vi "LoadItemValuesFromFile.vi"(0 "Array in":string[][](array[string]), 11 "error in (no error)":errorcluster) -> (3 "Values":dbl[](array[numeric]), 4 "Item":string, 6 "ZoomAlarmArray":dbl[][](array[numeric]), 8 "TimeString":string[](array[string]), 10 "TimeStamp":dbl[](array[numeric]), 13 "AlarmChannelNames":string[](array[string]), 14 "AlarmWaveforms":waveform(dbl)[](array[waveform]), 15 "error out":errorcluster)   [LabVIEW 2018]
doc: "Each row of the input string array specifies the Item, Dataset, Group, and Filepath of the data to be queried.\nUse these strings to look up the relevant data within the HDF5 records. The output values and corresponding TimeString or Timestamp arrays are suitable for plotting.\n\nItem (MaxValue, PeakLoc, etc.)\nDataset (Beac, Cal, etc.)\nGroup (84GHz_Cross, 72GHz_Cross, etc.)\nFile (filename of the HDF5 file)"
uses:
  HDF5/AI_alarm_data_cluster.ctl
  HDF5/HDF5_TC_Errors.ctl
  HDF5/TC_Data_Structure.ctl
  HDF5/HDF5_ToneInfoClust.ctl
  <vilib>/addons/h5labview2/file/H5Fmode.ctl
  HDF5/lib_path_mod_20200519.vi
  <vilib>/addons/h5labview2/base/H5Equery.vi
  <vilib>/addons/h5labview2/dataset/H5Dread.llb/H5Dread.xnode
  <vilib>/addons/h5labview2/file/H5F.lvlib
  <vilib>/addons/h5labview2/group/H5G.lvlib
  <vilib>/addons/h5labview2/dataset/H5D.lvlib
panel:
  in  "HDF5_TCInfo":T1
  in  "TC_alarm":T2
  in  "AI_alarm_Clust":T3
  # "Item"
  # "Dataset"
  # "Group"
  # "Filepath"
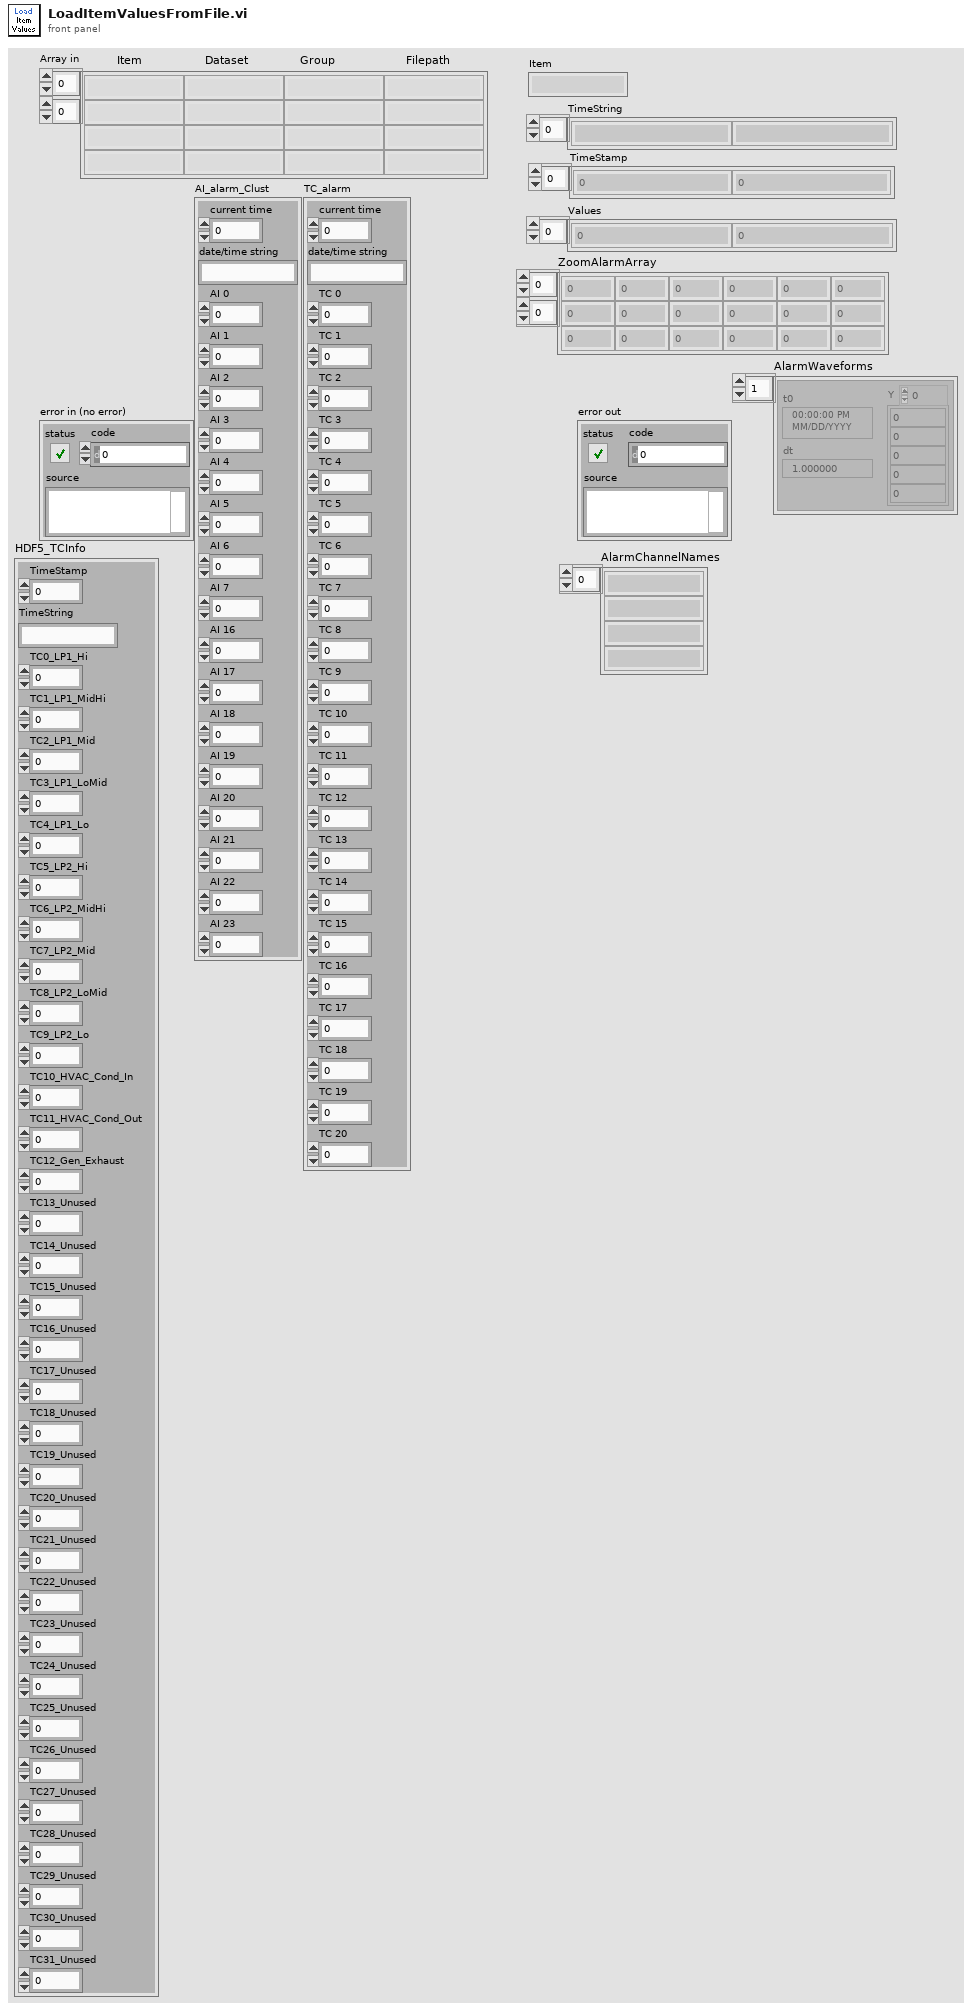
[diagram p1: front panel]
types:
  T1 = typedef "TC_Data_Structure.ctl" = cluster{"TimeStamp":dbl, "TimeString":string, "TC0_LP1_Hi":dbl, "TC1_LP1_MidHi":dbl, "TC2_LP1_Mid":dbl, "TC3_LP1_LoMid":dbl, "TC4_LP1_Lo":dbl, "TC5_LP2_Hi":dbl, "TC6_LP2_MidHi":dbl, "TC7_LP2_Mid":dbl, "TC8_LP2_LoMid":dbl, "TC9_LP2_Lo":dbl, "TC10_HVAC_Cond_In":dbl, "TC11_HVAC_Cond_Out":dbl, "TC12_Gen_Exhaust":dbl, "TC13_Unused":dbl, "TC14_Unused":dbl, "TC15_Unused":dbl, "TC16_Unused":dbl, "TC17_Unused":dbl, "TC18_Unused":dbl, "TC19_Unused":dbl, "TC20_Unused":dbl, "TC21_Unused":dbl, "TC22_Unused":dbl, "TC23_Unused":dbl, "TC24_Unused":dbl, "TC25_Unused":dbl, "TC26_Unused":dbl, "TC27_Unused":dbl, "TC28_Unused":dbl, "TC29_Unused":dbl, "TC30_Unused":dbl, "TC31_Unused":dbl}
  T2 = typedef "HDF5_TC_Errors.ctl" = cluster{"current time":dbl, "date/time string":string, "TC 0":dbl, "TC 1":dbl, "TC 2":dbl, "TC 3":dbl, "TC 4":dbl, "TC 5":dbl, "TC 6":dbl, "TC 7":dbl, "TC 8":dbl, "TC 9":dbl, "TC 10":dbl, "TC 11":dbl, "TC 12":dbl, "TC 13":dbl, "TC 14":dbl, "TC 15":dbl, "TC 16":dbl, "TC 17":dbl, "TC 18":dbl, "TC 19":dbl, "TC 20":dbl}
  T3 = typedef "AI_alarm_data_cluster.ctl" = cluster{"current time":dbl, "date/time string":string, "AI 0":dbl, "AI 1":dbl, "AI 2":dbl, "AI 3":dbl, "AI 4":dbl, "AI 5":dbl, "AI 6":dbl, "AI 7":dbl, "AI 16":dbl, "AI 17":dbl, "AI 18":dbl, "AI 19":dbl, "AI 20":dbl, "AI 21":dbl, "AI 22":dbl, "AI 23":dbl}
  T4 = typedef "H5F.lvlib/H5Fmode.ctl" = enum16{"read-only", "read-write", "overwrite", "create new", "open or create"}
  T5 = typedef "HDF5_ToneInfoClust.ctl" = cluster{"Timestring":string, "Timestamp":dbl, "MaxValue":dbl, "PeakLoc":dbl, "df":dbl}
  T6 = typedef "hid_t.ctl" = i32
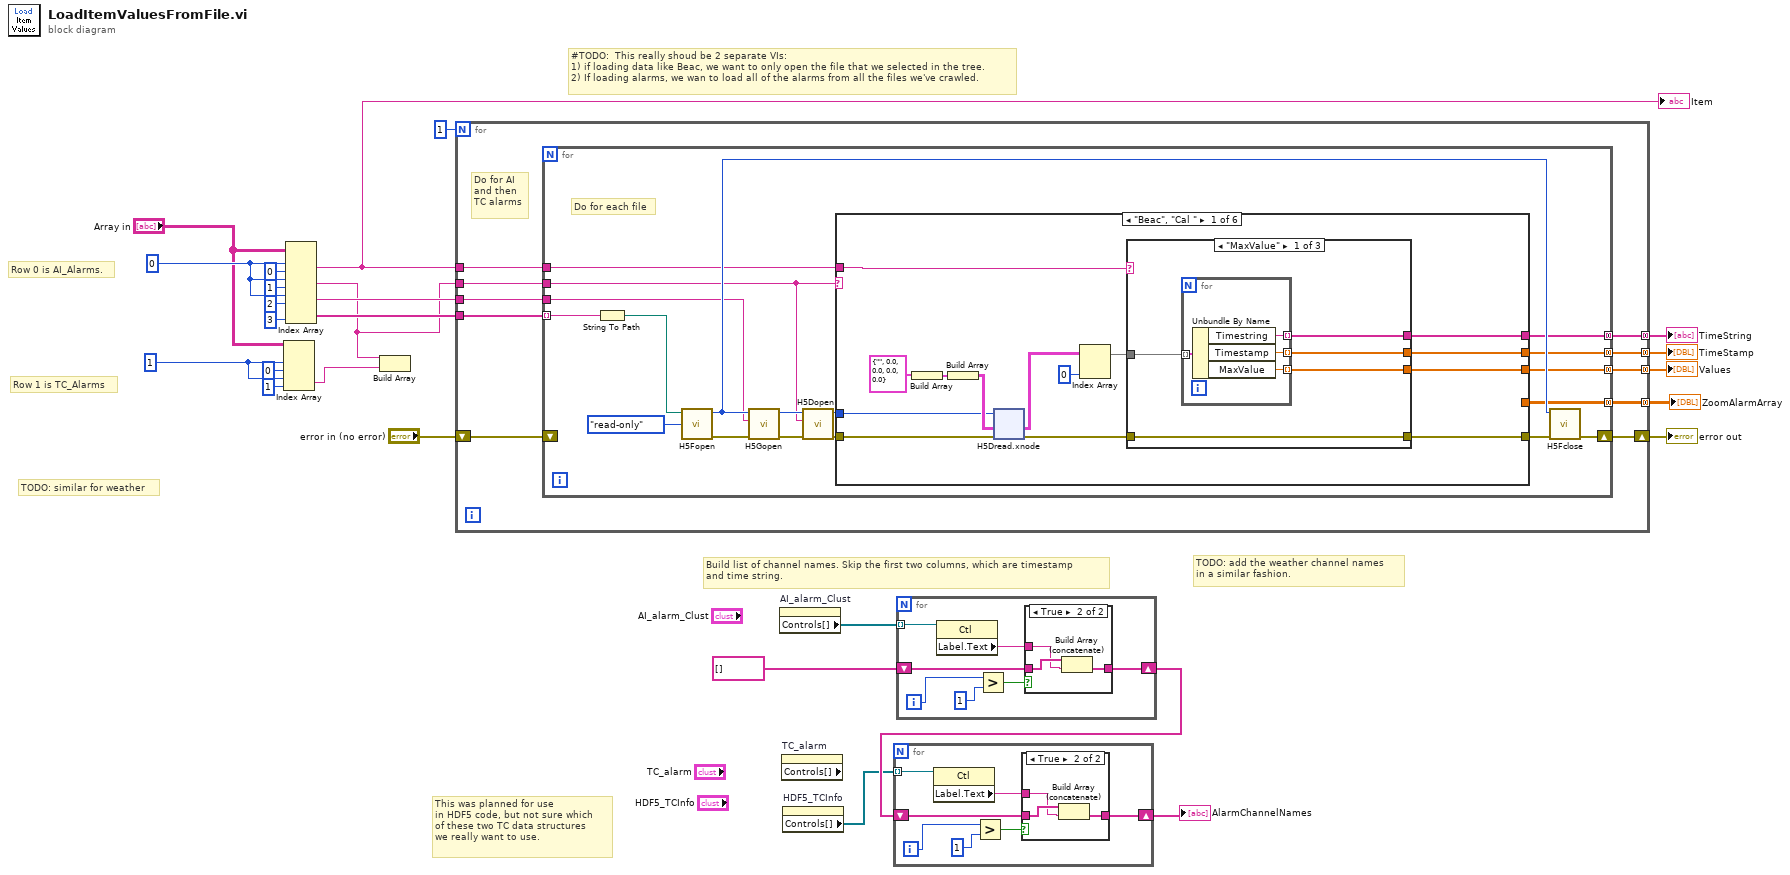
[diagram p0: block diagram]
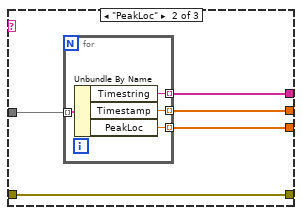
[diagram p2: hidden frame]
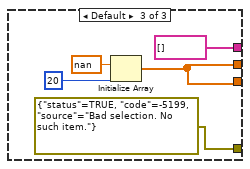
[diagram p3: hidden frame]
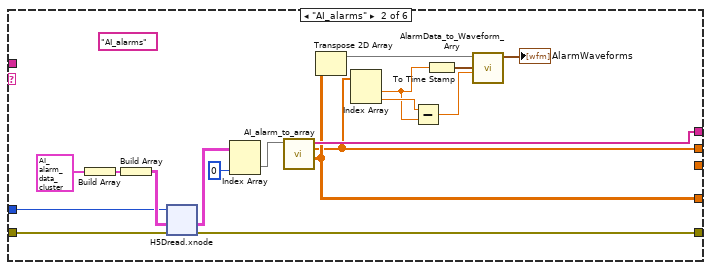
[diagram p4: hidden frame]
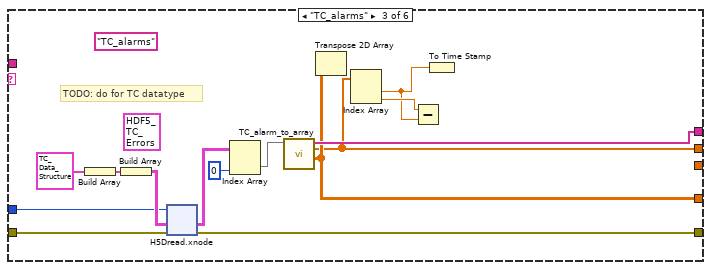
[diagram p5: hidden frame]
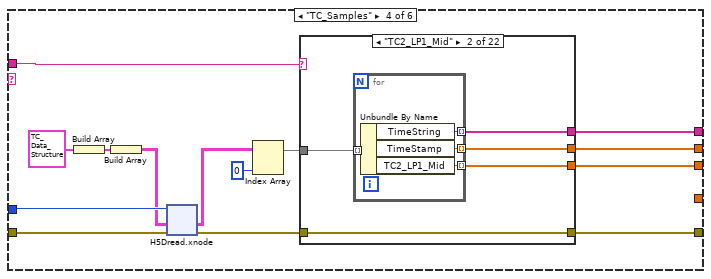
[diagram p6: hidden frame]
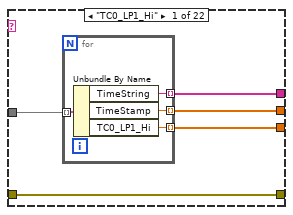
[diagram p7: hidden frame]
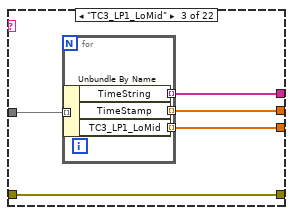
[diagram p8: hidden frame]
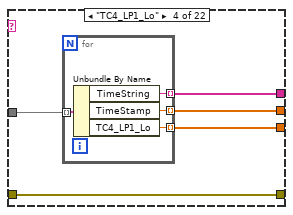
[diagram p9: hidden frame]
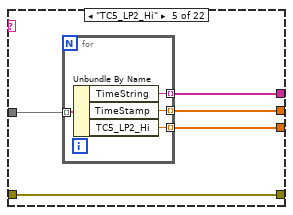
[diagram p10: hidden frame]
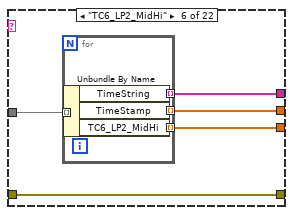
[diagram p11: hidden frame]
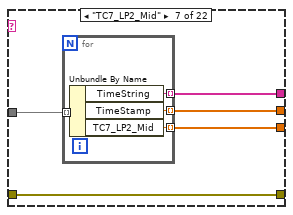
[diagram p12: hidden frame]
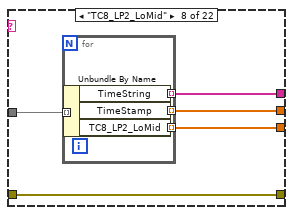
[diagram p13: hidden frame]
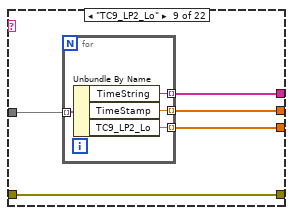
[diagram p14: hidden frame]
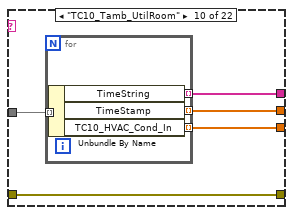
[diagram p15: hidden frame]
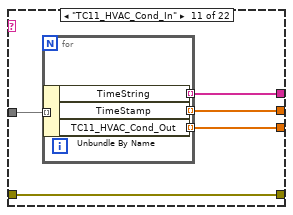
[diagram p16: hidden frame]
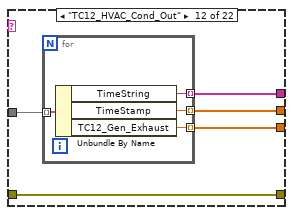
[diagram p17: hidden frame]
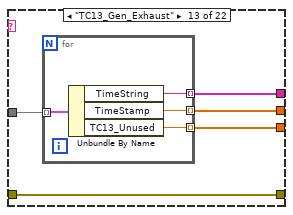
[diagram p18: hidden frame]
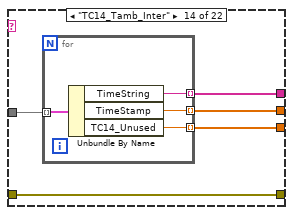
[diagram p19: hidden frame]
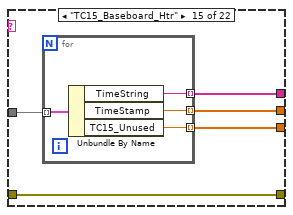
[diagram p20: hidden frame]
diagram:
  w5 = 1 ("disabled index (row)")
  w17 = 0 ("disabled index (row)")
  # "#TODO:  This really shoud be 2 separate VIs:\n1) if loading data like Beac, we want to only open the file that we selected in the tree.\n2) If loading alarms, we wan to load all of the alarms from all the files we've crawled."
  # "This was planned for use\nin HDF5 code, but not sure which\nof these two TC data structures\nwe really want to use."
  # "TODO: similar for weather"
  # "Row 1 is TC_Alarms"
  # "Row 0 is AI_Alarms."
  # "TODO: add the weather channel names\nin a similar fashion."
  # "Build list of channel names. Skip the first two columns, which are timestamp\nand time string."
  n1 = Index Array(array="Array in", index (row) #1=w5, index (col) #1=0 ("disabled index (col)"), index (row) #2=w5, index (col) #2=1 ("index (col)")) -> (element #2=w4:string)  [unwired: 1 out]
  n2 = Index Array(array="Array in", index (row) #1=w17, index (col) #1=0 ("disabled index (col)"), index (row) #2=w17, index (col) #2=1 ("index (col)"), index (row) #3=w17, index (col) #3=2 ("index (col)"), index (col) #4=3 ("index (row)")) -> (element #1=w24:string, element #2=w2:string, element #3=w19:string, element #4=w18:string[])  [unwired: 1 in]
  "Item" <- w24
  n3 = Build Array(w2, w4) -> ()  [unwired: 1 out]
  n4 = for {
    N: 1 -> [_]
    tunnel: w24 -> [w34]
    tunnel: [w33] -> w23 mode=concatenating
    tunnel: [w32] -> w22 mode=concatenating
    tunnel: [w31] -> w21 mode=concatenating
    tunnel: w19 -> [w30]
    tunnel: w18 -> [w29]
    tunnel: w2 -> [w28]
    tunnel: [w27] -> w13 mode=concatenating
    shift-right: [w35] -> w25
    shift-left: "error in (no error)" -> [w36]
    # "Do for AI\nand then \nTC alarms"
    n5 = for {
      tunnel: w29 -> [w52] mode=indexing
      tunnel: w34 -> [w42]
      tunnel: w28 -> [w43]
      tunnel: w30 -> [w44]
      tunnel: [w41] -> w31 mode=concatenating
      tunnel: [w40] -> w32 mode=concatenating
      tunnel: [w39] -> w33 mode=concatenating
      shift-right: [w38] -> w35
      shift-left: w36 -> [_]
      tunnel: [w37] -> w27 mode=concatenating
      # "Do for each file"
      n6 = String To Path(string=w52) -> (path=w51:path)
      n7 = call <vilib>:"H5Fopen.vi"("mode (read-only)"=H5Fmode."read-only" ("mode"), "path"=w51) -> ("error out"=w47:errorcluster, "ref out"=w45:T6)  [unwired: 8 in]
      n8 = call <vilib>:"H5Gopen.vi"("error in (no error)"=w47, "name"=w44, "ref in"=w45) -> ("error out"=w48:errorcluster, "group out"=w50:T6)  [unwired: 7 in]
      n9 = call <vilib>:"H5Dopen.vi"("error in (no error)"=w48, "name"=w43, "loc in"=w50) -> ("error out"=w46:errorcluster, "dset out"=w49:T6)  [unwired: 7 in]
      n10 = case shown="\"Beac\", \"Cal \"" w43 {
        tunnel: [w56 w117 w146 w170 w396 errorcluster {"status"=TRUE, "code"=-5198, "source"="Bad selection. No such group."} ("error out")] -> w53
        tunnel: w49 -> [w65 w122 w151 w182 w404 _]
        tunnel: w46 -> [w64 w121 w150 w181 w403 _]
        tunnel: w42 -> [w62 _ _ w179 w402 _]
        tunnel: [w59 w112 w143 w176 w397 w427] -> w41
        tunnel: [w58 _ _ w175 w398 w427] -> w40
        tunnel: [w55 w116 w145 w169 w394 string[] []] -> w39
        tunnel: [_ w115 w144 _ w392 _] -> w37
        frame "Beac", "Cal " {
          n11 = Build Array(T5 {"Timestring"="", "Timestamp"=0.0, "MaxValue"=0.0, "PeakLoc"=0.0, "df"=0.0} ("HDF5_ToneInfo in")) -> (w68:T5[])
          n12 = Build Array(w68) -> (w67:T5[][])
          n13 = xnode "H5Dread.xnode"("error in (no error)"=w64, "default"=w67, "ref in"=w65) -> ("error out"=w57:errorcluster, "data"=w63:T5[][])  [unwired: 3 in, 2 out]
          n14 = Index Array(array=w63, index (col)=0 ("disabled index (col)")) -> (element=w61:T5[])  [unwired: 1 in]
          n15 = case shown="\"MaxValue\"" w62 {
            tunnel: w61 -> [w73 w82 _]
            tunnel: [w72 w81 w89] -> w59
            tunnel: [w71 w80 w89] -> w58
            tunnel: w57 -> [w70 w79 _]
            tunnel: [w70 w79 errorcluster {"status"=TRUE, "code"=-5199, "source"="Bad selection. No such item."} ("error out")] -> w56
            tunnel: [w69 w78 string[] []] -> w55
            frame "MaxValue" {
              n16 = for {
                tunnel: w73 -> [w77] mode=indexing
                tunnel: [w76] -> w69 mode=indexing
                tunnel: [w75] -> w72 mode=indexing
                tunnel: [w74] -> w71 mode=indexing
                n17 = Unbundle By Name(w77) -> ("Timestring"=w76:string, "Timestamp"=w75:dbl, "MaxValue"=w74:dbl)
              }
            }
            frame "PeakLoc" {
              n18 = for {
                tunnel: w82 -> [w86] mode=indexing
                tunnel: [w85] -> w78 mode=indexing
                tunnel: [w84] -> w81 mode=indexing
                tunnel: [w83] -> w80 mode=indexing
                n19 = Unbundle By Name(w86) -> ("Timestring"=w85:string, "Timestamp"=w84:dbl, "PeakLoc"=w83:dbl)
              }
            }
            frame Default {
              n20 = Initialize Array(nan ("element"), 20 ("dimension size")) -> (w89:dbl[])
            }
          }
        }
        frame "AI_alarms" {
          (unwired) "AI_alarms" ("string")
          n21 = Build Array(T3 {"current time"=0.0, "date/time string"="", "AI 0"=0.0, "AI 1"=0.0, "AI 2"=0.0, "AI 3"=0.0, "AI 4"=0.0, "AI 5"=0.0, "AI 6"=0.0, "AI 7"=0.0, "AI 16"=0.0, "AI 17"=0.0, "AI 18"=0.0, "AI 19"=0.0, "AI 20"=0.0, "AI 21"=0.0, "AI 22"=0.0, "AI 23"=0.0} ("AI_alarm_Clust")) -> (w124:T3[])
          n22 = Build Array(w124) -> (w123:T3[][])
          n23 = xnode "H5Dread.xnode"("error in (no error)"=w121, "default"=w123, "ref in"=w122) -> ("error out"=w117:errorcluster, "data"=w120:T3[][])  [unwired: 3 in, 2 out]
          n24 = Index Array(array=w120, index (col)=0 ("disabled index (col)")) -> (element=w119:T3[])  [unwired: 1 in]
          n25 = call "AI_alarm_to_array.vi"("AI_alarms"=w119) -> ("AI_channel_data"=w115:dbl[][], "TimeStamp"=w112:dbl[], "TimeString"=w116:string[])  [unwired: 8 in]
          n26 = Transpose 2D Array(2D array=w115) -> (transposed array=w113:dbl[][])
          n27 = Index Array(array=w112) -> (element #1=w109:dbl, element #2=w110:dbl)  [unwired: 2 in]
          n28 = Subtract(x=w110, y=w109) -> (x-y=w108:dbl)
          n29 = To Time Stamp(1:w109) -> (0:w111:timestamp)
          n30 = call "AlarmData_to_Waveform_Arry.vi"("dt"=w108, "t0"=w111, "AI_channel_data"=w113) -> ("Array"=→"AlarmWaveforms":waveform(dbl)[])  [unwired: 8 in]
        }
        frame "TC_alarms" {
          (unwired) T2 {"current time"=0.0, "date/time string"="", "TC 0"=0.0, "TC 1"=0.0, "TC 2"=0.0, "TC 3"=0.0, "TC 4"=0.0, "TC 5"=0.0, "TC 6"=0.0, "TC 7"=0.0, "TC 8"=0.0, "TC 9"=0.0, "TC 10"=0.0, "TC 11"=0.0, "TC 12"=0.0, "TC 13"=0.0, "TC 14"=0.0, "TC 15"=0.0, "TC 16"=0.0, "TC 17"=0.0, "TC 18"=0.0, "TC 19"=0.0, "TC 20"=0.0} ("TC_alarm")
          (unwired) "TC_alarms" ("string")
          # "TODO: do for TC datatype"
          n31 = Build Array(T1 {"TimeStamp"=0.0, "TimeString"="", "TC0_LP1_Hi"=0.0, "TC1_LP1_MidHi"=0.0, "TC2_LP1_Mid"=0.0, "TC3_LP1_LoMid"=0.0, "TC4_LP1_Lo"=0.0, "TC5_LP2_Hi"=0.0, "TC6_LP2_MidHi"=0.0, "TC7_LP2_Mid"=0.0, "TC8_LP2_LoMid"=0.0, "TC9_LP2_Lo"=0.0, "TC10_HVAC_Cond_In"=0.0, "TC11_HVAC_Cond_Out"=0.0, "TC12_Gen_Exhaust"=0.0, "TC13_Unused"=0.0, "TC14_Unused"=0.0, "TC15_Unused"=0.0, "TC16_Unused"=0.0, "TC17_Unused"=0.0, "TC18_Unused"=0.0, "TC19_Unused"=0.0, "TC20_Unused"=0.0, "TC21_Unused"=0.0, "TC22_Unused"=0.0, "TC23_Unused"=0.0, "TC24_Unused"=0.0, "TC25_Unused"=0.0, "TC26_Unused"=0.0, "TC27_Unused"=0.0, "TC28_Unused"=0.0, "TC29_Unused"=0.0, "TC30_Unused"=0.0, "TC31_Unused"=0.0} ("HDF5_TCInfo")) -> (w153:T1[])
          n32 = Build Array(w153) -> (w152:T1[][])
          n33 = xnode "H5Dread.xnode"("error in (no error)"=w150, "default"=w152, "ref in"=w151) -> ("error out"=w146:errorcluster, "data"=w149:T1[][])  [unwired: 3 in, 2 out]
          n34 = Index Array(array=w149, index (col)=0 ("disabled index (col)")) -> (element=w148:T1[])  [unwired: 1 in]
          n35 = call "TC_alarm_to_array.vi"("TC_alarms"=w148) -> ("TC_channel_data"=w144:dbl[][], "TimeStamp"=w143:dbl[], "TimeString"=w145:string[])  [unwired: 8 in]
          n36 = Transpose 2D Array(2D array=w144) -> ()  [unwired: 1 out]
          n37 = Index Array(array=w143) -> (element #1=w141:dbl, element #2=w142:dbl)  [unwired: 2 in]
          n38 = Subtract(x=w142, y=w141) -> ()  [unwired: 1 out]
          n39 = To Time Stamp(1:w141) -> ()  [unwired: 1 out]
        }
        frame "TC_Samples" {
          n40 = Build Array(T1 {"TimeStamp"=0.0, "TimeString"="", "TC0_LP1_Hi"=0.0, "TC1_LP1_MidHi"=0.0, "TC2_LP1_Mid"=0.0, "TC3_LP1_LoMid"=0.0, "TC4_LP1_Lo"=0.0, "TC5_LP2_Hi"=0.0, "TC6_LP2_MidHi"=0.0, "TC7_LP2_Mid"=0.0, "TC8_LP2_LoMid"=0.0, "TC9_LP2_Lo"=0.0, "TC10_HVAC_Cond_In"=0.0, "TC11_HVAC_Cond_Out"=0.0, "TC12_Gen_Exhaust"=0.0, "TC13_Unused"=0.0, "TC14_Unused"=0.0, "TC15_Unused"=0.0, "TC16_Unused"=0.0, "TC17_Unused"=0.0, "TC18_Unused"=0.0, "TC19_Unused"=0.0, "TC20_Unused"=0.0, "TC21_Unused"=0.0, "TC22_Unused"=0.0, "TC23_Unused"=0.0, "TC24_Unused"=0.0, "TC25_Unused"=0.0, "TC26_Unused"=0.0, "TC27_Unused"=0.0, "TC28_Unused"=0.0, "TC29_Unused"=0.0, "TC30_Unused"=0.0, "TC31_Unused"=0.0} ("HDF5_TCInfo")) -> (w174:T1[])
          n41 = Build Array(w174) -> (w172:T1[][])
          n42 = xnode "H5Dread.xnode"("error in (no error)"=w181, "default"=w172, "ref in"=w182) -> ("error out"=w171:errorcluster, "data"=w180:T1[][])  [unwired: 3 in, 2 out]
          n43 = Index Array(array=w180, index (col)=0 ("disabled index (col)")) -> (element=w178:T1[])  [unwired: 1 in]
          n44 = case shown="\"TC2_LP1_Mid\"" w179 {
            tunnel: w178 -> [w187 w196 w205 w214 w223 w232 w241 w250 w259 w268 w277 w286 w295 w304 w313 w322 w331 w340 w349 w358 w367 _]
            tunnel: [w186 w195 w204 w213 w222 w231 w240 w249 w258 w267 w276 w285 w294 w303 w312 w321 w330 w339 w348 w357 w366 w374] -> w176
            tunnel: [w185 w194 w203 w212 w221 w230 w239 w248 w257 w266 w275 w284 w293 w302 w311 w320 w329 w338 w347 w356 w365 w374] -> w175
            tunnel: w171 -> [w184 w193 w202 w211 w220 w229 w238 w247 w256 w265 w274 w283 w292 w301 w310 w319 w328 w337 w346 w355 w364 _]
            tunnel: [w184 w193 w202 w211 w220 w229 w238 w247 w256 w265 w274 w283 w292 w301 w310 w319 w328 w337 w346 w355 w364 errorcluster {"status"=TRUE, "code"=-5199, "source"="Bad selection. No such item."} ("error out")] -> w170
            tunnel: [w183 w192 w201 w210 w219 w228 w237 w246 w255 w264 w273 w282 w291 w300 w309 w318 w327 w336 w345 w354 w363 string[] []] -> w169
            frame "TC0_LP1_Hi" {
              n45 = for {
                tunnel: w187 -> [w191] mode=indexing
                tunnel: [w190] -> w183 mode=indexing
                tunnel: [w189] -> w186 mode=indexing
                tunnel: [w188] -> w185 mode=indexing
                n46 = Unbundle By Name(w191) -> ("TimeString"=w190:string, "TimeStamp"=w189:dbl, "TC0_LP1_Hi"=w188:dbl)
              }
            }
            frame "TC2_LP1_Mid" {
              n47 = for {
                tunnel: w196 -> [w200] mode=indexing
                tunnel: [w199] -> w192 mode=indexing
                tunnel: [w198] -> w195 mode=indexing
                tunnel: [w197] -> w194 mode=indexing
                n48 = Unbundle By Name(w200) -> ("TimeString"=w199:string, "TimeStamp"=w198:dbl, "TC2_LP1_Mid"=w197:dbl)
              }
            }
            frame "TC3_LP1_LoMid" {
              n49 = for {
                tunnel: w205 -> [w209] mode=indexing
                tunnel: [w208] -> w201 mode=indexing
                tunnel: [w207] -> w204 mode=indexing
                tunnel: [w206] -> w203 mode=indexing
                n50 = Unbundle By Name(w209) -> ("TimeString"=w208:string, "TimeStamp"=w207:dbl, "TC3_LP1_LoMid"=w206:dbl)
              }
            }
            frame "TC4_LP1_Lo" {
              n51 = for {
                tunnel: w214 -> [w218] mode=indexing
                tunnel: [w217] -> w210 mode=indexing
                tunnel: [w216] -> w213 mode=indexing
                tunnel: [w215] -> w212 mode=indexing
                n52 = Unbundle By Name(w218) -> ("TimeString"=w217:string, "TimeStamp"=w216:dbl, "TC4_LP1_Lo"=w215:dbl)
              }
            }
            frame "TC5_LP2_Hi" {
              n53 = for {
                tunnel: w223 -> [w227] mode=indexing
                tunnel: [w226] -> w219 mode=indexing
                tunnel: [w225] -> w222 mode=indexing
                tunnel: [w224] -> w221 mode=indexing
                n54 = Unbundle By Name(w227) -> ("TimeString"=w226:string, "TimeStamp"=w225:dbl, "TC5_LP2_Hi"=w224:dbl)
              }
            }
            frame "TC6_LP2_MidHi" {
              n55 = for {
                tunnel: w232 -> [w236] mode=indexing
                tunnel: [w235] -> w228 mode=indexing
                tunnel: [w234] -> w231 mode=indexing
                tunnel: [w233] -> w230 mode=indexing
                n56 = Unbundle By Name(w236) -> ("TimeString"=w235:string, "TimeStamp"=w234:dbl, "TC6_LP2_MidHi"=w233:dbl)
              }
            }
            frame "TC7_LP2_Mid" {
              n57 = for {
                tunnel: w241 -> [w245] mode=indexing
                tunnel: [w244] -> w237 mode=indexing
                tunnel: [w243] -> w240 mode=indexing
                tunnel: [w242] -> w239 mode=indexing
                n58 = Unbundle By Name(w245) -> ("TimeString"=w244:string, "TimeStamp"=w243:dbl, "TC7_LP2_Mid"=w242:dbl)
              }
            }
            frame "TC8_LP2_LoMid" {
              n59 = for {
                tunnel: w250 -> [w254] mode=indexing
                tunnel: [w253] -> w246 mode=indexing
                tunnel: [w252] -> w249 mode=indexing
                tunnel: [w251] -> w248 mode=indexing
                n60 = Unbundle By Name(w254) -> ("TimeString"=w253:string, "TimeStamp"=w252:dbl, "TC8_LP2_LoMid"=w251:dbl)
              }
            }
            frame "TC9_LP2_Lo" {
              n61 = for {
                tunnel: w259 -> [w263] mode=indexing
                tunnel: [w262] -> w255 mode=indexing
                tunnel: [w261] -> w258 mode=indexing
                tunnel: [w260] -> w257 mode=indexing
                n62 = Unbundle By Name(w263) -> ("TimeString"=w262:string, "TimeStamp"=w261:dbl, "TC9_LP2_Lo"=w260:dbl)
              }
            }
            frame "TC10_Tamb_UtilRoom" {
              n63 = for {
                tunnel: w268 -> [w272] mode=indexing
                tunnel: [w271] -> w264 mode=indexing
                tunnel: [w270] -> w267 mode=indexing
                tunnel: [w269] -> w266 mode=indexing
                n64 = Unbundle By Name(w272) -> ("TimeString"=w271:string, "TimeStamp"=w270:dbl, "TC10_HVAC_Cond_In"=w269:dbl)
              }
            }
            frame "TC11_HVAC_Cond_In" {
              n65 = for {
                tunnel: w277 -> [w281] mode=indexing
                tunnel: [w280] -> w273 mode=indexing
                tunnel: [w279] -> w276 mode=indexing
                tunnel: [w278] -> w275 mode=indexing
                n66 = Unbundle By Name(w281) -> ("TimeString"=w280:string, "TimeStamp"=w279:dbl, "TC11_HVAC_Cond_Out"=w278:dbl)
              }
            }
            frame "TC12_HVAC_Cond_Out" {
              n67 = for {
                tunnel: w286 -> [w290] mode=indexing
                tunnel: [w289] -> w282 mode=indexing
                tunnel: [w288] -> w285 mode=indexing
                tunnel: [w287] -> w284 mode=indexing
                n68 = Unbundle By Name(w290) -> ("TimeString"=w289:string, "TimeStamp"=w288:dbl, "TC12_Gen_Exhaust"=w287:dbl)
              }
            }
            frame "TC13_Gen_Exhaust" {
              n69 = for {
                tunnel: w295 -> [w299] mode=indexing
                tunnel: [w298] -> w291 mode=indexing
                tunnel: [w297] -> w294 mode=indexing
                tunnel: [w296] -> w293 mode=indexing
                n70 = Unbundle By Name(w299) -> ("TimeString"=w298:string, "TimeStamp"=w297:dbl, "TC13_Unused"=w296:dbl)
              }
            }
            frame "TC14_Tamb_Inter" {
              n71 = for {
                tunnel: w304 -> [w308] mode=indexing
                tunnel: [w307] -> w300 mode=indexing
                tunnel: [w306] -> w303 mode=indexing
                tunnel: [w305] -> w302 mode=indexing
                n72 = Unbundle By Name(w308) -> ("TimeString"=w307:string, "TimeStamp"=w306:dbl, "TC14_Unused"=w305:dbl)
              }
            }
            frame "TC15_Baseboard_Htr" {
              n73 = for {
                tunnel: w313 -> [w317] mode=indexing
                tunnel: [w316] -> w309 mode=indexing
                tunnel: [w315] -> w312 mode=indexing
                tunnel: [w314] -> w311 mode=indexing
                n74 = Unbundle By Name(w317) -> ("TimeString"=w316:string, "TimeStamp"=w315:dbl, "TC15_Unused"=w314:dbl)
              }
            }
            frame "TC16_CPU_Rack" {
              n75 = for {
                tunnel: w322 -> [w326] mode=indexing
                tunnel: [w325] -> w318 mode=indexing
                tunnel: [w324] -> w321 mode=indexing
                tunnel: [w323] -> w320 mode=indexing
                n76 = Unbundle By Name(w326) -> ("TimeString"=w325:string, "TimeStamp"=w324:dbl, "TC16_Unused"=w323:dbl)
              }
            }
            frame "TC17_Antenna_Rear" {
              n77 = for {
                tunnel: w331 -> [w335] mode=indexing
                tunnel: [w334] -> w327 mode=indexing
                tunnel: [w333] -> w330 mode=indexing
                tunnel: [w332] -> w329 mode=indexing
                n78 = Unbundle By Name(w335) -> ("TimeString"=w334:string, "TimeStamp"=w333:dbl, "TC17_Unused"=w332:dbl)
              }
            }
            frame "TC18_Tamb_GlobeLo" {
              n79 = for {
                tunnel: w340 -> [w344] mode=indexing
                tunnel: [w343] -> w336 mode=indexing
                tunnel: [w342] -> w339 mode=indexing
                tunnel: [w341] -> w338 mode=indexing
                n80 = Unbundle By Name(w344) -> ("TimeString"=w343:string, "TimeStamp"=w342:dbl, "TC18_Unused"=w341:dbl)
              }
            }
            frame "TC19_Tamb_GlobeHi" {
              n81 = for {
                tunnel: w349 -> [w353] mode=indexing
                tunnel: [w352] -> w345 mode=indexing
                tunnel: [w351] -> w348 mode=indexing
                tunnel: [w350] -> w347 mode=indexing
                n82 = Unbundle By Name(w353) -> ("TimeString"=w352:string, "TimeStamp"=w351:dbl, "TC19_Unused"=w350:dbl)
              }
            }
            frame "TC20_InvertChargeOut " {
              n83 = for {
                tunnel: w358 -> [w362] mode=indexing
                tunnel: [w361] -> w354 mode=indexing
                tunnel: [w360] -> w357 mode=indexing
                tunnel: [w359] -> w356 mode=indexing
                n84 = Unbundle By Name(w362) -> ("TimeString"=w361:string, "TimeStamp"=w360:dbl, "TC20_Unused"=w359:dbl)
              }
            }
            frame "TC1_LP1_MidHi" {
              n85 = for {
                tunnel: w367 -> [w371] mode=indexing
                tunnel: [w370] -> w363 mode=indexing
                tunnel: [w369] -> w366 mode=indexing
                tunnel: [w368] -> w365 mode=indexing
                n86 = Unbundle By Name(w371) -> ("TimeString"=w370:string, "TimeStamp"=w369:dbl, "TC1_LP1_MidHi"=w368:dbl)
              }
            }
            frame Default {
              n87 = Initialize Array(nan ("element"), 20 ("dimension size")) -> (w374:dbl[])
            }
          }
        }
        frame "BeacZoom", "CalZoom" {
          # "This should be 2D array. Ex:\n54434x20"
          n88 = Build Array(dbl[] [0.0, 0.0, 0.0, 0.0, 0.0, 0.0, 0.0, 0.0, 0.0, 0.0, 0.0, 0.0, 0.0, 0.0, 0.0, 0.0, 0.0, 0.0, 0.0, 0.0, 0.0, 0.0, 0.0, 0.0, 0.0, 0.0, 0.0, 0.0, 0.0, 0.0, 0.0, 0.0, 0.0, 0.0, 0.0, 0.0, 0.0, 0.0, 0.0, 0.0, 0.0, 0.0, 0.0, 0.0, 0.0, 0.0, 0.0, 0.0, 0.0, 0.0, 0.0, 0.0, 0.0, 0.0, 0.0, 0.0, 0.0, 0.0, 0.0, 0.0, 0.0, 0.0, 0.0, 0.0, 0.0, 0.0, 0.0, 0.0, 0.0, 0.0, 0.0, 0.0, 0.0, 0.0, 0.0, 0.0, 0.0, 0.0, 0.0, 0.0, 0.0, 0.0, 0.0, 0.0, 0.0, 0.0, 0.0, 0.0, 0.0, 0.0, 0.0, 0.0, 0.0, 0.0, 0.0, 0.0, 0.0, 0.0, 0.0, 0.0, 0.0, 0.0, 0.0, 0.0, 0.0, 0.0, 0.0, 0.0, 0.0, 0.0, 0.0, 0.0, 0.0, 0.0, 0.0, 0.0, 0.0, 0.0, 0.0, 0.0, 0.0, 0.0, 0.0, 0.0, 0.0, 0.0, 0.0, 0.0, 0.0, 0.0, 0.0, 0.0, 0.0, 0.0, 0.0, 0.0, 0.0, 0.0, 0.0, 0.0, 0.0, 0.0, 0.0, 0.0, 0.0, 0.0, 0.0, 0.0, 0.0, 0.0, 0.0, 0.0, 0.0, 0.0, 0.0, 0.0, 0.0, 0.0, 0.0, 0.0, 0.0, 0.0, 0.0, 0.0, 0.0, 0.0, 0.0, 0.0, 0.0, 0.0, 0.0, 0.0, 0.0, 0.0, 0.0, 0.0, 0.0, 0.0, 0.0, 0.0, 0.0, 0.0, 0.0, 0.0, 0.0, 0.0, 0.0, 0.0, 0.0, 0.0, 0.0, 0.0, 0.0, 0.0, 0.0, 0.0, 0.0, 0.0, 0.0, 0.0, 0.0, 0.0, 0.0, 0.0, 0.0, 0.0, 0.0, 0.0, 0.0, 0.0, 0.0, 0.0, 0.0, 0.0, 0.0, 0.0, 0.0, 0.0, 0.0, 0.0, 0.0, 0.0, 0.0, 0.0, 0.0, 0.0, 0.0, 0.0, 0.0, 0.0, 0.0, 0.0, 0.0, 0.0, 0.0, 0.0, 0.0, 0.0, 0.0, 0.0, 0.0, 0.0, 0.0, 0.0, 0.0, 0.0, 0.0, 0.0, 0.0, 0.0, 0.0, 0.0, 0.0, 0.0, 0.0, 0.0, 0.0, 0.0, 0.0, 0.0, 0.0, 0.0, 0.0, 0.0, 0.0, 0.0, 0.0, 0.0, 0.0, 0.0, 0.0, 0.0, 0.0, 0.0, 0.0, 0.0, 0.0, 0.0, 0.0, 0.0, 0.0, 0.0, 0.0, 0.0, 0.0, 0.0, 0.0, 0.0, 0.0, 0.0, 0.0, 0.0, 0.0, 0.0, 0.0, 0.0, 0.0, 0.0, 0.0, 0.0, 0.0, 0.0, 0.0, 0.0, 0.0, 0.0, 0.0, 0.0, 0.0, 0.0, 0.0, 0.0, 0.0, 0.0, 0.0, 0.0, 0.0, 0.0, 0.0, 0.0, 0.0, 0.0, 0.0, 0.0, 0.0, 0.0, 0.0, 0.0, 0.0, 0.0, 0.0, 0.0, 0.0, 0.0, 0.0, 0.0, 0.0, 0.0, 0.0, 0.0, 0.0, 0.0, 0.0, 0.0, 0.0, 0.0, 0.0, 0.0, 0.0, 0.0, 0.0, 0.0, 0.0, 0.0, 0.0, 0.0, 0.0, 0.0, 0.0, 0.0, 0.0, 0.0, 0.0, 0.0, 0.0, 0.0, 0.0, 0.0, 0.0, 0.0, 0.0, 0.0, 0.0, 0.0, 0.0, 0.0, 0.0, 0.0, 0.0, 0.0, 0.0, 0.0, 0.0, 0.0, 0.0, 0.0, 0.0, 0.0, 0.0, 0.0, 0.0, 0.0, 0.0, 0.0, 0.0, 0.0, 0.0, 0.0, 0.0, 0.0, 0.0, 0.0, 0.0, 0.0, 0.0, 0.0, 0.0, 0.0, 0.0, 0.0, 0.0, 0.0, 0.0, 0.0, 0.0, 0.0, 0.0, 0.0, 0.0, 0.0, 0.0, 0.0, 0.0, 0.0, 0.0, 0.0, 0.0, 0.0, 0.0, 0.0, 0.0, 0.0, 0.0, 0.0, 0.0, 0.0, 0.0, 0.0, 0.0, 0.0, 0.0, 0.0, 0.0, 0.0, 0.0, 0.0, 0.0, 0.0, 0.0, 0.0, 0.0, 0.0, 0.0, 0.0, 0.0, 0.0, 0.0, 0.0, 0.0, 0.0, 0.0, 0.0, 0.0, 0.0, 0.0, 0.0, 0.0, 0.0, 0.0, 0.0, 0.0, 0.0, 0.0, 0.0, 0.0, 0.0, 0.0, 0.0, 0.0, 0.0, 0.0, 0.0, 0.0, 0.0, 0.0, 0.0, 0.0, 0.0, 0.0, 0.0, 0.0, 0.0, 0.0, 0.0, 0.0, 0.0, 0.0, 0.0, 0.0, 0.0, 0.0, 0.0, 0.0, 0.0, 0.0, 0.0, 0.0, 0.0, 0.0, 0.0, 0.0, 0.0, 0.0, 0.0, 0.0, 0.0, 0.0, 0.0, 0.0, 0.0, 0.0, 0.0, 0.0, 0.0, 0.0, 0.0, 0.0, 0.0, 0.0, 0.0, 0.0, 0.0, 0.0, 0.0, 0.0, 0.0, 0.0, 0.0, 0.0, 0.0, 0.0, 0.0, 0.0, 0.0, 0.0, 0.0, 0.0, 0.0, 0.0, 0.0, 0.0, 0.0, 0.0, 0.0, 0.0, 0.0, 0.0, 0.0, 0.0, 0.0, 0.0, 0.0, 0.0, 0.0, 0.0, 0.0, 0.0, 0.0, 0.0, 0.0, 0.0, 0.0, 0.0, 0.0, 0.0, 0.0, 0.0, 0.0, 0.0, 0.0, 0.0, 0.0, 0.0, 0.0, 0.0, 0.0, 0.0, 0.0, 0.0, 0.0, 0.0, 0.0, 0.0, 0.0, 0.0, 0.0, 0.0, 0.0, 0.0, 0.0, 0.0, 0.0, 0.0, 0.0, 0.0, 0.0, 0.0, 0.0, 0.0, 0.0, 0.0, 0.0, 0.0, 0.0, 0.0, 0.0, 0.0, 0.0, 0.0, 0.0, 0.0, 0.0, 0.0, 0.0, 0.0, 0.0, 0.0, 0.0, 0.0, 0.0, 0.0, 0.0, 0.0, 0.0, 0.0, 0.0, 0.0, 0.0, 0.0, 0.0, 0.0, 0.0, 0.0, 0.0, 0.0, 0.0, 0.0, 0.0, 0.0, 0.0, 0.0, 0.0, 0.0, 0.0, 0.0, 0.0, 0.0, 0.0, 0.0, 0.0, 0.0, 0.0, 0.0, 0.0, 0.0, 0.0, 0.0, 0.0, 0.0, 0.0, 0.0, 0.0, 0.0, 0.0, 0.0, 0.0, 0.0, 0.0, 0.0, 0.0, 0.0, 0.0, 0.0, 0.0, 0.0, 0.0, 0.0, 0.0, 0.0, 0.0, 0.0, 0.0, 0.0, 0.0, 0.0, 0.0, 0.0, 0.0, 0.0, 0.0, 0.0, 0.0, 0.0, 0.0, 0.0, 0.0, 0.0, 0.0, 0.0, 0.0, 0.0, 0.0, 0.0, 0.0, 0.0, 0.0, 0.0, 0.0, 0.0, 0.0, 0.0, 0.0, 0.0, 0.0, 0.0, 0.0, 0.0, 0.0, 0.0, 0.0, 0.0, 0.0, 0.0, 0.0, 0.0, 0.0, 0.0, 0.0, 0.0, 0.0, 0.0, 0.0, 0.0, 0.0, 0.0, 0.0, 0.0, 0.0, 0.0, 0.0, 0.0, 0.0, 0.0, 0.0, 0.0, 0.0, 0.0, 0.0, 0.0, 0.0, 0.0, 0.0, 0.0, 0.0, 0.0, 0.0, 0.0, 0.0, 0.0, 0.0, 0.0, 0.0, 0.0, 0.0, 0.0, 0.0, 0.0, 0.0, 0.0, 0.0, 0.0, 0.0, 0.0, 0.0, 0.0, 0.0, 0.0, 0.0, 0.0, 0.0, 0.0, 0.0, 0.0, 0.0, 0.0, 0.0, 0.0, 0.0, 0.0, 0.0, 0.0, 0.0, 0.0, 0.0, 0.0, 0.0, 0.0, 0.0, 0.0, 0.0, 0.0, 0.0, 0.0, 0.0, 0.0, 0.0, 0.0, 0.0, 0.0, 0.0, 0.0, 0.0, 0.0, 0.0, 0.0, 0.0, 0.0, 0.0, 0.0, 0.0, 0.0, 0.0, 0.0, 0.0, 0.0, 0.0, 0.0, 0.0, 0.0, 0.0, 0.0, 0.0, 0.0, 0.0, 0.0, 0.0, 0.0, 0.0, 0.0, 0.0, 0.0, 0.0, 0.0, 0.0, 0.0, 0.0, 0.0, 0.0, 0.0, 0.0, 0.0, 0.0, 0.0, 0.0, 0.0, 0.0, 0.0, 0.0, 0.0, 0.0, 0.0, 0.0, 0.0, 0.0, 0.0, 0.0, 0.0, 0.0, 0.0, 0.0, 0.0, 0.0, 0.0, 0.0, 0.0, 0.0, 0.0, 0.0, 0.0, 0.0, 0.0, 0.0, 0.0, 0.0, 0.0, 0.0, 0.0, 0.0, 0.0, 0.0, 0.0, 0.0, 0.0, 0.0, 0.0, 0.0, 0.0, 0.0, 0.0, 0.0, 0.0, 0.0, 0.0, 0.0, 0.0, 0.0, 0.0, 0.0, 0.0, 0.0, 0.0, 0.0, 0.0, 0.0, 0.0, 0.0, 0.0, 0.0, 0.0, 0.0, 0.0, 0.0, 0.0, 0.0, 0.0, 0.0, 0.0, 0.0, 0.0, 0.0, 0.0, 0.0, 0.0, 0.0, 0.0, 0.0, 0.0, 0.0, 0.0, 0.0, 0.0, 0.0, 0.0, 0.0, 0.0, 0.0, 0.0, 0.0, 0.0, 0.0, 0.0, 0.0, 0.0, 0.0, 0.0, 0.0, 0.0, 0.0, 0.0, 0.0, 0.0, 0.0, 0.0, 0.0, 0.0, 0.0, 0.0, 0.0, 0.0, 0.0, 0.0, 0.0, 0.0, 0.0, 0.0, 0.0, 0.0, 0.0, 0.0, 0.0, 0.0, 0.0, 0.0, 0.0, 0.0, 0.0, 0.0, 0.0, 0.0, 0.0, 0.0, 0.0, 0.0, 0.0, 0.0, 0.0, 0.0, 0.0, 0.0, 0.0, 0.0, 0.0, 0.0, 0.0, 0.0, 0.0, 0.0, 0.0, 0.0, 0.0, 0.0, 0.0, 0.0, 0.0] ("Zoom")) -> (w405:dbl[][])
          n89 = xnode "H5Dread.xnode"("error in (no error)"=w403, "default"=w405, "ref in"=w404) -> ("error out"=w395:errorcluster, "data"=w393:dbl[][])  [unwired: 3 in, 2 out]
          n90 = Index Array(array=w393, index (col)=0 ("disabled index (col)")) -> (element=w401:dbl[])  [unwired: 1 in]
          n91 = case shown="Default" w402 {
            tunnel: w401 -> [w410]
            tunnel: [w410] -> w398
            tunnel: [dbl[] [] ("Zoom")] -> w397
            tunnel: [w409] -> w396
            tunnel: w395 -> [w409]
            tunnel: [string[] []] -> w394
            tunnel: w393 -> [w406]
            tunnel: [w406] -> w392
            frame Default {
            }
          }
        }
        frame Default {
          n92 = Initialize Array(nan ("element"), 20 ("dimension size")) -> (w427:dbl[])
        }
      }
      n93 = call <vilib>:"H5Fclose.vi"("error in (no error)"=w53, "ref"=w45) -> ("error out"=w38:errorcluster)  [unwired: 9 in]
    }
  }
  "error out" <- w25
  "TimeString" <- w23
  "Values" <- w22
  "TimeStamp" <- w21
  "ZoomAlarmArray" <- w13
  n94 = property on="AI_alarm_Clust" class="Clust (strict)"() -> ("Controls[]"=w12:refnum<vi>[])  [unwired: 2 in, 2 out]
  n95 = property on="TC_alarm" class="Clust (strict)" props=["Controls[]"]() -> ()  [unwired: 2 in, 3 out]
  n96 = property on="HDF5_TCInfo" class="Clust (strict)"() -> ("Controls[]"=w3:refnum<vi>[])  [unwired: 2 in, 2 out]
  n97 = for {
    tunnel: w12 -> [w437] mode=indexing
    shift-right: [w431] -> w9
    shift-left: string[] [] -> [w432]
    i -> [w435]
    n98 = property class="Ctl"(reference=w437) -> ("Label.Text"=w433:string)  [unwired: 1 in, 2 out]
    n99 = Greater?(x=w435, y=1) -> (0:w436:bool)
    n100 = case shown="True" w436 {
      tunnel: w433 -> [_ w439]
      tunnel: w432 -> [w438 w440]
      tunnel: [w438 w441] -> w431
      frame False {
      }
      frame True {
        n101 = Build Array (concatenate)(w440, w439) -> (w441:string[])
      }
    }
  }
  n102 = for {
    tunnel: w3 -> [w448] mode=indexing
    shift-right: [w442] -> w10
    shift-left: w9 -> [w443]
    i -> [w446]
    n103 = property class="Ctl"(reference=w448) -> ("Label.Text"=w444:string)  [unwired: 1 in, 2 out]
    n104 = Greater?(x=w446, y=1) -> (0:w447:bool)
    n105 = case shown="True" w447 {
      tunnel: w444 -> [_ w450]
      tunnel: w443 -> [w449 w451]
      tunnel: [w449 w452] -> w442
      frame False {
      }
      frame True {
        n106 = Build Array (concatenate)(w451, w450) -> (w452:string[])
      }
    }
  }
  "AlarmChannelNames" <- w10
